vi "FPGA_Dental robot output c.vi"() -> ()   [LabVIEW 2018]
uses:
  <vilib>/Platform/TimedLoop/XDataNode/timing_clust.ctl
  <vilib>/Platform/TimedLoop/XDataNode/nitl_modes.ctl
  <vilib>/Platform/TimedLoop/XDataNode/wakeup.ctl
  <vilib>/rvi/Emulation/niFpgaGetClockAttributes.vi
  <vilib>/rvi/Emulation/niFpgaSctlEmulationGetInTimedLoop.vi
  <vilib>/rvi/Emulation/niFpgaEmulationReportErrorSimple.vi
  <vilib>/rvi/Emulation/niFpgaProcessEmulError.vi
  <vilib>/rvi/eio/common/nirviEmuTemplateMethod_errors.vi
  <vilib>/rvi/Emulation/niFpgaCriticalErrorInLSC.vi
  <vilib>/eio/EIONode/EIONode.xnode
  <vilib>/Platform/TimedLoop/XDataNode/XDataNode.xnode
  <vilib>/Platform/TimedLoop/XDataNode/XDNodeRunTimeDep.lvlib
panel:
  out "C4":bool
  out "C3":bool
  out "C2":bool
  out "C1":bool
  in  "B/AO1":u16
  in  "B/AO0":u16
  in  "A/AO1":u16
  in  "A/AO0":u16
  out "Channel1":u16
  out "Channel2":u16
  out "Channel3":u16
  out "Channel4":u16
  in  "stop":bool
  in  "DIR4":bool
  in  "ENA4":bool
  in  "STBY4":bool
  out "JumpBy2Error 4":i16
  in  "CH4 DC":fxp<+,32,0>
  out "Position4":i32
  in  "Reset 4":bool
  in  "DIR3":bool
  in  "ENA3":bool
  in  "STBY3":bool
  out "JumpBy2Error 3":i16
  in  "CH3 DC":fxp<+,32,0>
  out "Position3":i32
  in  "Reset 3":bool
  in  "DIR2":bool
  in  "ENA2":bool
  in  "STBY2":bool
  out "JumpBy2Error 2":i16
  in  "CH2 DC":fxp<+,32,0>
  out "Position2":i32
  in  "Reset 2":bool
  in  "Reset 1":bool
  out "Position1":i32
  in  "CH1 DC":fxp<+,32,0>
  out "JumpBy2Error 1":i16
  in  "STBY1":bool
  in  "ENA1":bool
  in  "DIR1":bool
  # "Motor control"
  # "Current feedback"
  # "Channel 1"
  # "Channel 2"
  # "Channel 3"
  # "Channel 4"
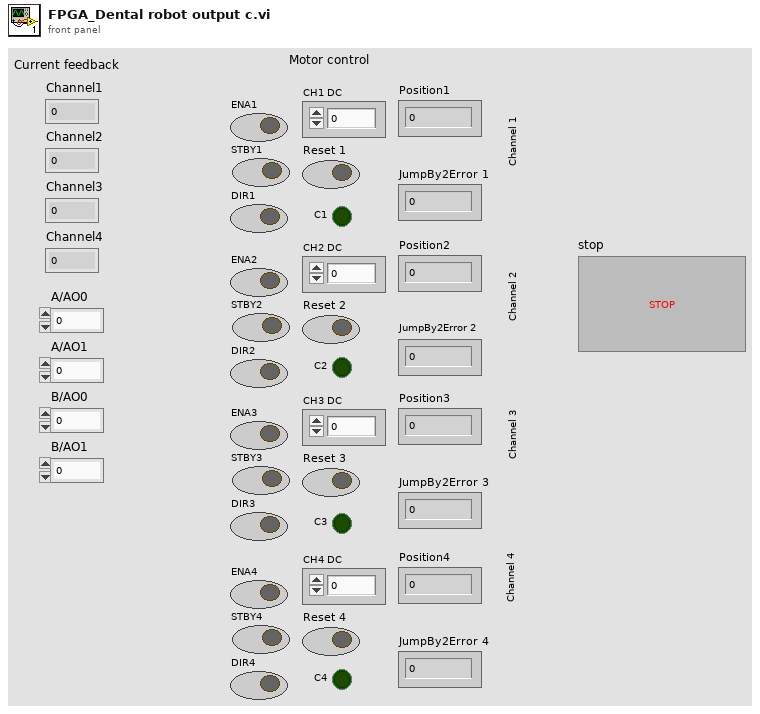
[diagram p1: front panel]
types:
  T1 = cluster{"FPGA I/O":refnum<k21>, "FPGA I/O 2":refnum<k21>, "FPGA I/O 3":refnum<k21>, "FPGA I/O 4":refnum<k21>, "FPGA I/O 5":refnum<k21>, "FPGA I/O 6":refnum<k21>, "FPGA I/O 7":refnum<k21>}
  T2 = typedef "XDNodeRunTimeDep.lvlib/timing_clust.ctl" = cluster{"Expected End [f-1]":u64, "Actual End [f-1]":u64, "Finished Late? [f-1]":bool, "Expected End [i-1]":u64, "Actual End [i-1]":u64, "Finished Late? [i-1]":bool, "Expected Start [i]":u64, "Actual Start [i]":u64, "Expected Start [f]":u64, "Actual Start [f]":u64, "Source Name":string, "Structure Name":string, "Period":i64, "Deadline":i64, "Offset":i64, "Start":i64, "Priority":i32, "Timeout":i32, "Mode":T3, "Wakeup Reason":T4, "Error":errorcluster, "Source Type":string, "Secondary Source Type":string, "Global End Time":u64, "Global Start Time":u64, "Frame Duration":u64, "Iteration Duration":u64, "Assigned CPU":i32, "I/O Scan Engine Mode":u32}
  T3 = typedef "XDNodeRunTimeDep.lvlib/nitl_modes.ctl" = enum32{"No Change", "Process missed periods, maintain original phase", "Discard missed periods, maintain original phase", "Process missed periods, ignore original phase", "Discard missed periods, ignore original phase"}
  T4 = typedef "XDNodeRunTimeDep.lvlib/wakeup.ctl" = enum32{"Normal", "Aborted", "Asynchronous wakeup", "Timing source error", "Timed loop error", "Timeout"}
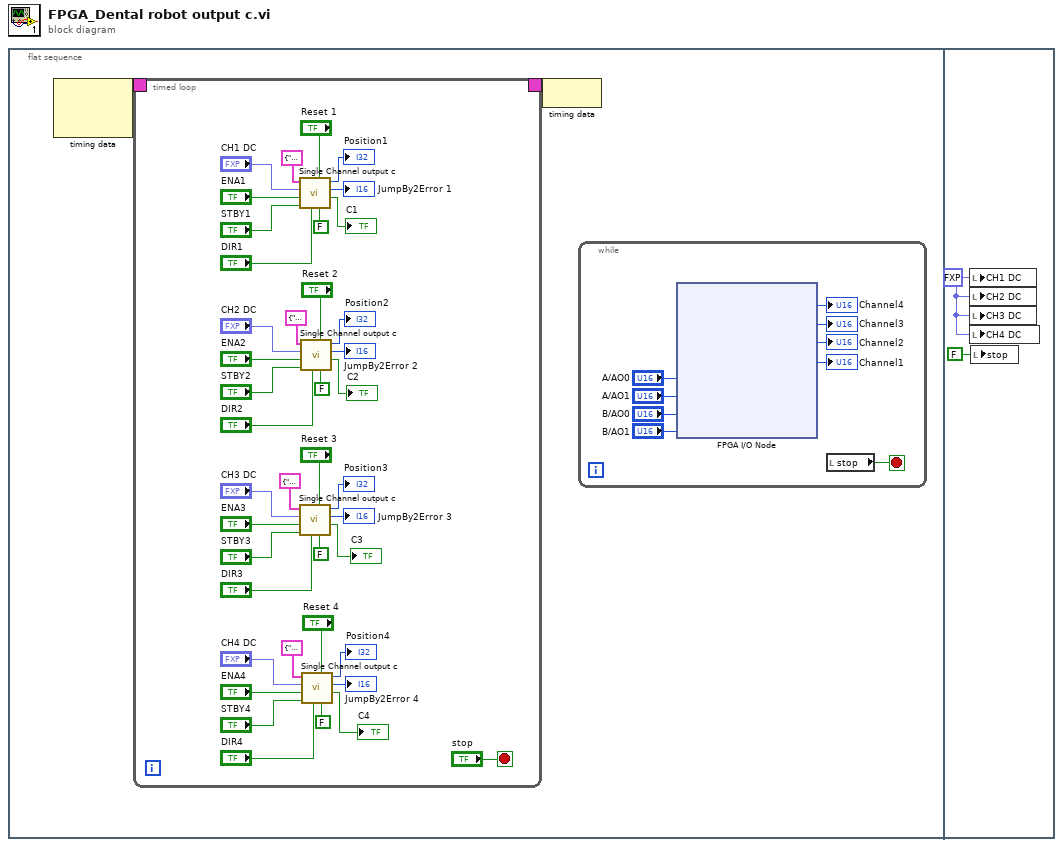
[diagram p0: block diagram]
diagram:
  n1 = flat-sequence {
    frame #0 {
      n2 = node-c288() -> (w2:T2)  [unwired: 2 in]
      n3 = timed-loop {
        timing: w2 -> [_]
        timing-out: [_] -> w1
        stop <- "stop" stop-if-true
        n4 = call "Single Channel output c.vi"("Reset by Enc C"=FALSE, "Reset by hand"="Reset 1", "DIR"="DIR1", "STBY"="STBY1", "ENA"="ENA1", "Duty"="CH1 DC", "I/O Channel"=T1 {"FPGA I/O"="ConnectorA/DIO6", "FPGA I/O 2"="ConnectorA/DIO5", "FPGA I/O 3"="ConnectorA/DIO4", "FPGA I/O 4"="ConnectorA/DIO3", "FPGA I/O 5"="ConnectorA/DIO2", "FPGA I/O 6"="ConnectorA/DIO1", "FPGA I/O 7"="ConnectorA/DIO0"}) -> ("C"=→"C1":bool, "JumpBy2Error"=→"JumpBy2Error 1":i16, "Position"=→"Position1":i32)  [unwired: 2 in]
        n5 = call "Single Channel output c.vi"("Reset by Enc C"=FALSE, "Reset by hand"="Reset 3", "DIR"="DIR3", "STBY"="STBY3", "ENA"="ENA3", "Duty"="CH3 DC", "I/O Channel"=T1 {"FPGA I/O"="ConnectorB/DIO6", "FPGA I/O 2"="ConnectorB/DIO5", "FPGA I/O 3"="ConnectorB/DIO4", "FPGA I/O 4"="ConnectorB/DIO3", "FPGA I/O 5"="ConnectorB/DIO2", "FPGA I/O 6"="ConnectorB/DIO1", "FPGA I/O 7"="ConnectorB/DIO0"}) -> ("C"=→"C3":bool, "JumpBy2Error"=→"JumpBy2Error 3":i16, "Position"=→"Position3":i32)  [unwired: 2 in]
        n6 = call "Single Channel output c.vi"("Reset by Enc C"=FALSE, "Reset by hand"="Reset 2", "DIR"="DIR2", "STBY"="STBY2", "ENA"="ENA2", "Duty"="CH2 DC", "I/O Channel"=T1 {"FPGA I/O"="ConnectorA/DIO13", "FPGA I/O 2"="ConnectorA/DIO12", "FPGA I/O 3"="ConnectorA/DIO11", "FPGA I/O 4"="ConnectorA/DIO10", "FPGA I/O 5"="ConnectorA/DIO9", "FPGA I/O 6"="ConnectorA/DIO8", "FPGA I/O 7"="ConnectorA/DIO7"}) -> ("C"=→"C2":bool, "JumpBy2Error"=→"JumpBy2Error 2":i16, "Position"=→"Position2":i32)  [unwired: 2 in]
        n7 = call "Single Channel output c.vi"("Reset by Enc C"=FALSE, "Reset by hand"="Reset 4", "DIR"="DIR4", "STBY"="STBY4", "ENA"="ENA4", "Duty"="CH4 DC", "I/O Channel"=T1 {"FPGA I/O"="ConnectorB/DIO13", "FPGA I/O 2"="ConnectorB/DIO12", "FPGA I/O 3"="ConnectorB/DIO11", "FPGA I/O 4"="ConnectorB/DIO10", "FPGA I/O 5"="ConnectorB/DIO9", "FPGA I/O 6"="ConnectorB/DIO8", "FPGA I/O 7"="ConnectorB/DIO7"}) -> ("C"=→"C4":bool, "JumpBy2Error"=→"JumpBy2Error 4":i16, "Position"=→"Position4":i32)  [unwired: 2 in]
      }
      n8 = node-c288(w1) -> ()
      n9 = while {
        stop <- w3 stop-if-true
        n10 = xnode "FPGA I/O Node"("ConnectorA/AO0"="A/AO0", "ConnectorA/AO1"="A/AO1", "ConnectorB/AO0"="B/AO0", "ConnectorB/AO1"="B/AO1") -> ("ConnectorA/AI0"=→"Channel4":u16, "ConnectorA/AI1"=→"Channel3":u16, "ConnectorA/AI2"=→"Channel2":u16, "ConnectorA/AI3"=→"Channel1":u16)  [unwired: 8 in, 8 out]
        n11 = local read "stop"() -> (w3:bool)
      }
    }
    frame #1 {
      w58 = fxp<+,32,0> 0.0 ("CH1 DC")
      n12 = local write "CH1 DC"(w58) -> ()
      n13 = local write "CH2 DC"(w58) -> ()
      n14 = local write "CH3 DC"(w58) -> ()
      n15 = local write "CH4 DC"(w58) -> ()
      n16 = local write "stop"(FALSE ("stop")) -> ()
    }
  }
